vi "writePicoBatch.vi"(8 "error in (no error)":errorcluster, 9 "Raw Data Folder":path, 10 "File Name":string, 11 "Full Scan Name":string) -> (0 "error out":errorcluster)   [LabVIEW 2013]
panel:
  out "concatenated string":string
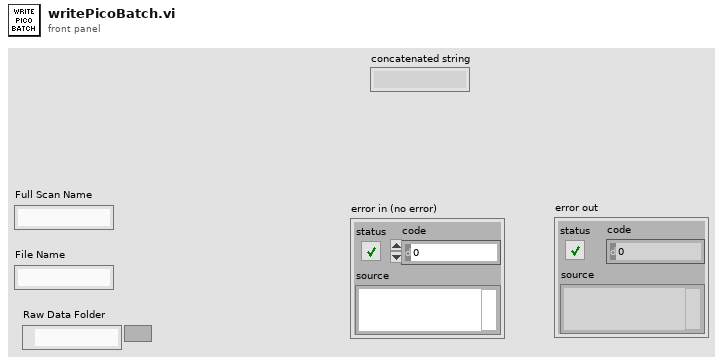
[diagram p1: front panel]
types:
  T1 = enum16{"open", "replace", "create", "open or create", "replace or create", "replace or create with confirmation"}
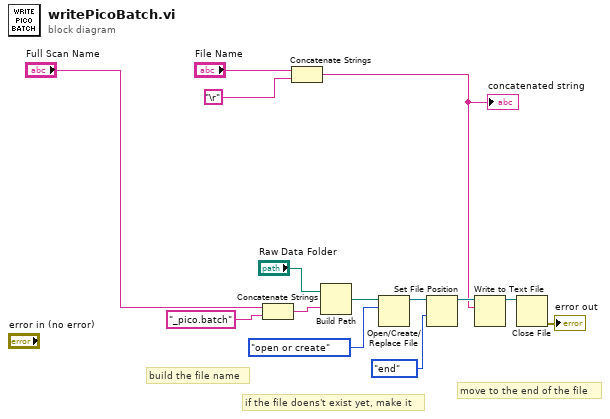
[diagram p0: block diagram]
diagram:
  # "move to the end of the file"
  # "if the file doens't exist yet, make it"
  # "build the file name"
  n1 = Concatenate Strings("Full Scan Name", "_pico.batch" ("string")) -> (w13:string)
  n2 = Concatenate Strings("File Name", "\r") -> (w2:string)
  "concatenated string" <- w2
  n3 = Build Path(base path="Raw Data Folder", name or relative path=w13) -> (appended path=w11:path)
  n4 = Open/Create/Replace File(file path (use dialog)=w11, operation (0:open)=T1."open or create") -> (refnum out=w7:refnum<file>)  [unwired: 4 in, 2 out]
  n5 = Set File Position(refnum=w7, from (0:start)=enum16{"start", "end", "current"}."end") -> (refnum out=w8:refnum<file>)  [unwired: 2 in, 1 out]
  n6 = Write to Text File(file (use dialog)=w8, text=w2) -> (refnum out=w9:refnum<file>)  [unwired: 2 in, 2 out]
  n7 = Close File(refnum=w9) -> (error out=→"error out":errorcluster)  [unwired: 1 in, 1 out]
